vi "ImageSimulator.vi"(1 "y_start":u32=1, 2 "x_start":u32=1, 3 "ImageCnt":u32=1, 4 "FilePath":string) -> ()   [LabVIEW 2012]
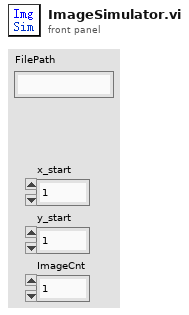
[diagram p1: front panel]
types:
  T1 = typedef "Image Type" = u32
  T2 = typedef "IMAQ Image.ctl" = refnum<image>
  T3 = cluster{"image":i16[][], "x_start":u32, "x_end":u32, "y_start":u32, "y_end":u32, "ImageCnt":u32, "subImage":u16[][]}
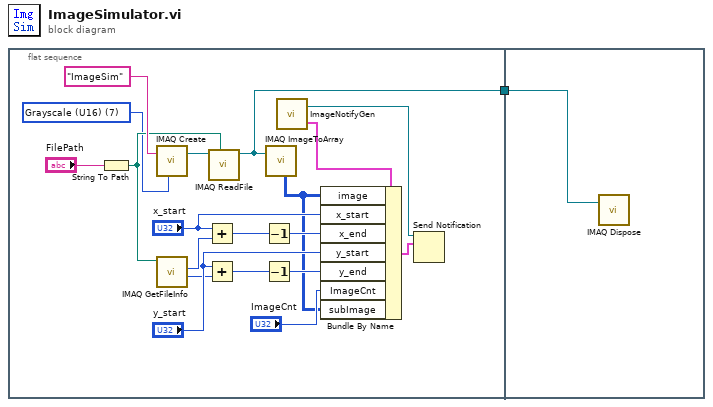
[diagram p0: block diagram]
diagram:
  n1 = flat-sequence {
    tunnel: [w3] -> w1
    tunnel: w1 -> [w21]
    frame #0 {
      w4 = T1 7 items=["Grayscale (U8)", "Grayscale (I16)", "Grayscale (SGL)", "Complex (CSG)", "RGB (U32)", "HSL (U32)", "RGB (U64)", "Grayscale (U16)"] ("Image Type")
      n2 = String To Path(string="FilePath") -> (path=w11:path)
      n3 = call "IMAQ Create"("Image Name"="ImageSim", "Image Type"=w4) -> ("New Image"=w13:T2)  [unwired: 3 in, 1 out]
      n4 = call "IMAQ GetFileInfo"("File Path"=w11) -> ("Y Resolution"=w9:i32, "X Resolution"=w10:i32)  [unwired: 4 in, 5 out]
      n5 = Add(x="x_start", y=w10) -> (x+y=w8:u32)
      n6 = Add(x="y_start", y=w9) -> (x+y=w6:u32)
      n7 = call "IMAQ ReadFile"("File Path"=w11, "Image"=w13) -> ("Image Out"=w3:T2)  [unwired: 5 in, 4 out]
      n8 = Decrement(x=w8) -> (x-1=w7:u32)
      n9 = Decrement(x=w6) -> (x-1=w5:u32)
      n10 = call "IMAQ ImageToArray"("Image"=w3) -> ("Image Pixels (U16)"=w2:u16[][])  [unwired: 3 in, 4 out]
      n11 = call "ImageNotifyGen.vi"() -> ("ImageClusterRef"=w20:T3, "ImageNotifyRef"=w19:refnum<notifier>)  [unwired: 2 in]
      n12 = Bundle By Name(cluster=w20, "image"=w2, "x_start"="x_start", "x_end"=w7, "y_start"="y_start", "y_end"=w5, "ImageCnt"="ImageCnt", "subImage"=w2) -> (w18:T3)
      n13 = Send Notification(notification=w18, notifier=w19) -> ()  [unwired: 1 in, 2 out]
    }
    frame #1 {
      n14 = call "IMAQ Dispose"("Image"=w21) -> ()  [unwired: 5 in, 1 out]
    }
  }
